vi "Generate Transformation Matrix.vi"(8 "error in":errorcluster, 11 "Referential in":refnum<class "Referential.lvclass">) -> (0 "error out":errorcluster, 2 "Matrix":T1, 3 "Referential out":refnum<class "Referential.lvclass">)   [LabVIEW 2019, in "Referential.lvclass"]
uses:
  Referential.lvclass
  <vilib>/Analysis/Matrix/Datatypes/RealMatrix.ctl
  <vilib>/Analysis/baseanly.llb/Real A x B.vi
  <vilib>/Analysis/Matrix/NI_Matrix.lvlib
  <vilib>/Analysis/NI_AALBase.lvlib
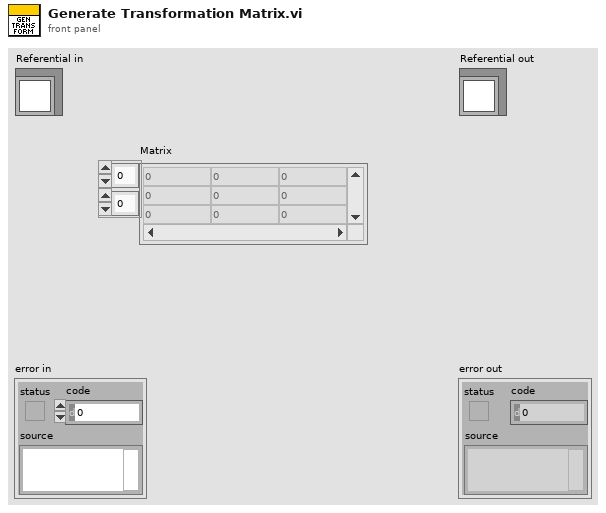
[diagram p1: front panel]
types:
  T1 = typedef "NI_Matrix.lvlib/RealMatrix.ctl" = dbl[][]
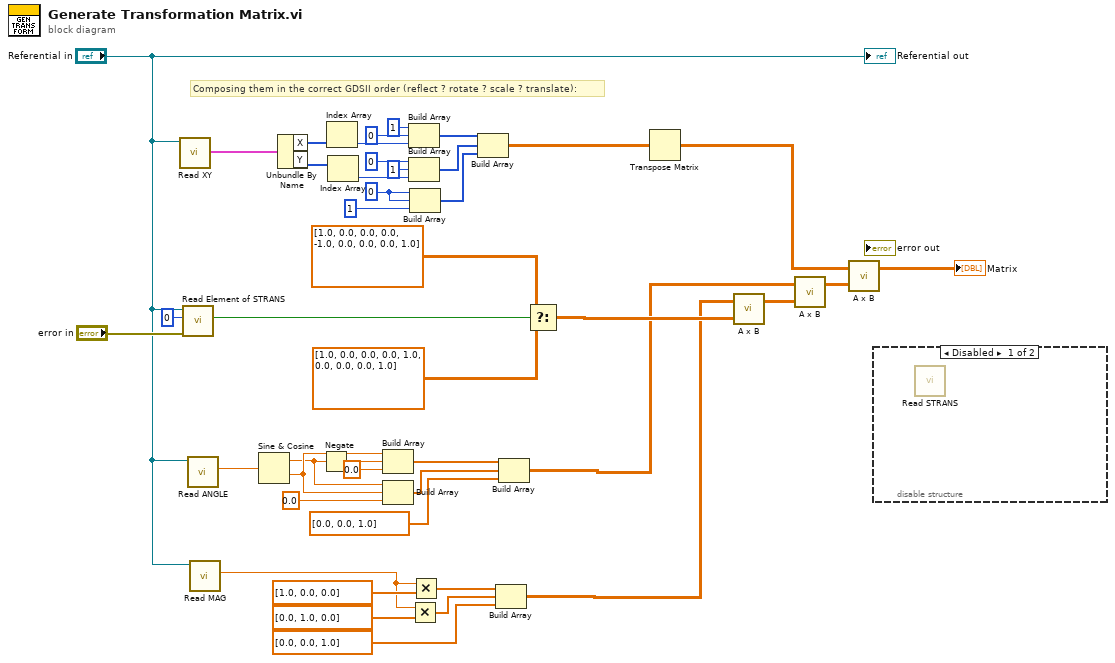
[diagram p0: block diagram]
diagram:
  w17 = 0 ("element")
  # "Composing them in the correct GDSII order (reflect ? rotate ? scale ? translate):"
  n1 = call-dynamic "Read XY.vi"("Element in"="Referential in") -> ("XY"=w22:cluster{"X":i32[], "Y":i32[]})  [unwired: 8 in, 2 out]
  n2 = call-dynamic "Read Element of STRANS.vi"("error in (no error)"="error in", "index"=0, "Referential in"="Referential in") -> ("Bit"=w34:bool)  [unwired: 6 in, 2 out]
  n3 = call-dynamic "Read ANGLE.vi"("Referential in"="Referential in") -> ("ANGLE"=w41:dbl)  [unwired: 8 in, 2 out]
  n4 = call-dynamic "Read MAG.vi"("Referential in"="Referential in") -> ("MAG"=w30:dbl)  [unwired: 8 in, 2 out]
  n5 = Sine & Cosine(0:w41) -> (1:w36:dbl, 2:w37:dbl)
  n6 = Unbundle By Name(w22) -> ("X"=w21:i32[], "Y"=w20:i32[])
  n7 = Negate(x=w36) -> (-x=w40:dbl)
  n8 = Index Array(array=w21) -> (element=w19:i32)  [unwired: 1 in]
  n9 = Index Array(array=w20) -> (element=w15:i32)  [unwired: 1 in]
  n10 = Build Array(w37, w40, 0.0 ("element")) -> (w35:dbl[])
  n11 = Build Array(w36, w37, 0.0 ("element")) -> (w27:dbl[])
  n12 = Build Array(1 ("element"), 0 ("element"), w19) -> (w11:i32[])
  n13 = Build Array(0 ("element"), 1 ("element"), w15) -> (w10:i32[])
  n14 = Build Array(w17, w17, 1 ("element")) -> (w9:i32[])
  n15 = Multiply(x=w30, y=dbl[] [0.0, 1.0, 0.0] ("element")) -> (x*y=w26:dbl[])
  n16 = Multiply(x=w30, y=dbl[] [1.0, 0.0, 0.0] ("element")) -> (x*y=w31:dbl[])
  n17 = Build Array(w11, w10, w9) -> (w2:T1)
  n18 = Build Array(w31, w26, dbl[] [0.0, 0.0, 1.0] ("element")) -> (w7:T1)
  n19 = Build Array(w35, w27, dbl[] [0.0, 0.0, 1.0] ("element")) -> (w5:T1)
  n20 = Select(t=T1 [[1.0, 0.0, 0.0], [0.0, -1.0, 0.0], [0.0, 0.0, 1.0]] ("appended array"), s=w34, f=T1 [[1.0, 0.0, 0.0], [0.0, 1.0, 0.0], [0.0, 0.0, 1.0]] ("appended array")) -> (s? t:f=w8:T1)
  n21 = Transpose Matrix(1:w2) -> (0:w1:T1)
  n22 = call-poly <vilib>:"A x B.vi"("B"=w8, "A"=w7) -> ("A x B"=w6:T1)  [unwired: 1 out]
  n23 = call-poly <vilib>:"A x B.vi"("B"=w6, "A"=w5) -> ("A x B"=w4:T1)  [unwired: 1 out]
  n24 = call-poly <vilib>:"A x B.vi"("B"=w4, "A"=w1) -> ("A x B"=→"Matrix":T1)  [unwired: 1 out]
  n25 = disable-structure shown="Disabled" {
    frame Disabled {
      n26 = call-dynamic "Read STRANS.vi"() -> ()  [unwired: 9 in, 3 out]
    }
    frame Enabled {
    }
  }
  "Referential out" <- "Referential in"
